vi "Led.vi"() -> ()   [LabVIEW 2020]
panel:
  in  "stop":bool
  out "Меньше нуля":bool
  out "Больше нуля":bool
  in  "Число":dbl
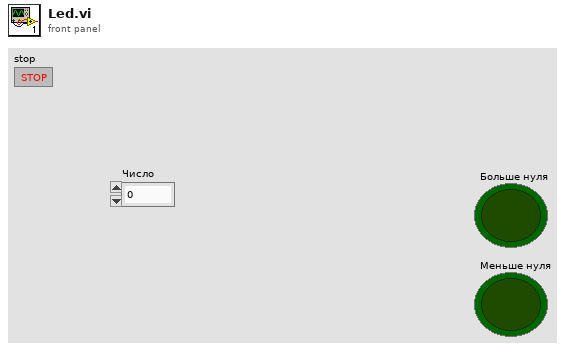
[diagram p1: front panel]
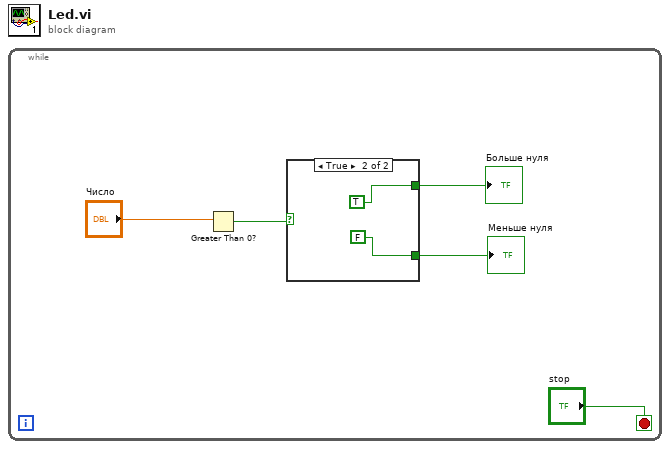
[diagram p0: block diagram]
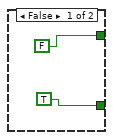
[diagram p2: hidden frame]
diagram:
  n1 = while {
    stop <- "stop" stop-if-true
    n2 = Greater Than 0?(x="Число") -> (x > 0?=w5:bool)
    n3 = case shown="True" w5 {
      tunnel: [TRUE FALSE] -> w3
      tunnel: [FALSE TRUE] -> w2
      frame False {
      }
      frame True {
      }
    }
    "Больше нуля" <- w2
    "Меньше нуля" <- w3
  }
